vi "Update_W_b.vi"(0 "W_l":T1, 1 "Learning_Rate":dbl, 2 "dW_l":T1, 3 "b_l":T1, 4 "db_l":T1) -> (5 "New_Wl":T1, 6 "New_bl":T1)   [LabVIEW 2016]
uses:
  <vilib>/Analysis/Matrix/Datatypes/RealMatrix.ctl
  <vilib>/Analysis/Matrix/Numeric/Multiply/Multiply - R,RM.vi
  <vilib>/Analysis/Matrix/Numeric/Subtract/Subtract - RM,RM.vi
  <vilib>/Analysis/Matrix/Numeric/Multiply/Multiply - RM,R.vi
  <vilib>/Analysis/Matrix/NI_Matrix.lvlib
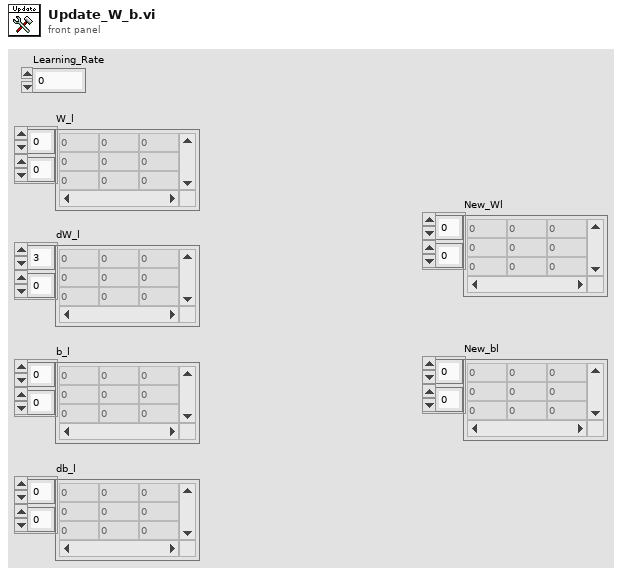
[diagram p1: front panel]
types:
  T1 = typedef "NI_Matrix.lvlib/RealMatrix.ctl" = dbl[][]
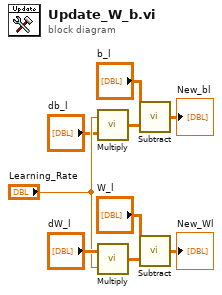
[diagram p0: block diagram]
diagram:
  n1 = call-poly <vilib>:"Multiply.vi"("Real Matrix A"="db_l", "Real Scalar c"="Learning_Rate") -> ("c * A"=w2:T1)
  n2 = call-poly <vilib>:"Multiply.vi"("Real Scalar c"="Learning_Rate", "Real Matrix A"="dW_l") -> ("A * c"=w5:T1)
  n3 = call-poly <vilib>:"Subtract.vi"("Real Matrix B"=w2, "Real Matrix A"="b_l") -> ("A - B"=→"New_bl":T1)
  n4 = call-poly <vilib>:"Subtract.vi"("Real Matrix B"=w5, "Real Matrix A"="W_l") -> ("A - B"=→"New_Wl":T1)
